vi "LinearQuadraticRegulator_Calculate.vi"(9 "X":T1, 11 "in LinearQuadraticRegulator":T2) -> (0 "Error":bool, 2 "U":T1, 3 "out LinearQuadraticRegulator":T2)   [LabVIEW 2019, in "Trajectory_Library.lvlib"]
doc: "Returns the next output of the controller.\n\nInputs:\n - LinearQuadraticRegulator -- controller data cluster \n - x -- The current state x.\n\nOutput:\n - outLinearQuadraticRegulator -- updated controller data cluster\n - U -- The next controller output.\n - error -- If TRUE, an error occured."
uses:
  Trajectory_Library.lvlib
  <vilib>/Analysis/NI_AALBase.lvlib
  <vilib>/Analysis/baseanly.llb/Real A x B.vi
  <vilib>/Analysis/Matrix/NI_Matrix.lvlib
  <vilib>/Analysis/Matrix/Numeric/Subtract/Subtract - RM,RM.vi
  <vilib>/Analysis/Matrix/Datatypes/RealMatrix.ctl
  TypeDef/LINEAR_QUADRATIC_REGULATOR.ctl
panel:
  # "Ref State <States,1>"
  # "Comp and capped \noutput <Inputs,1>"
  # "Controller gain\n<Inputs,States>"
  # "Ref State <States,1>"
  # "Comp and capped \noutput <Inputs,1>"
  # "Controller gain\n<Inputs,States>"
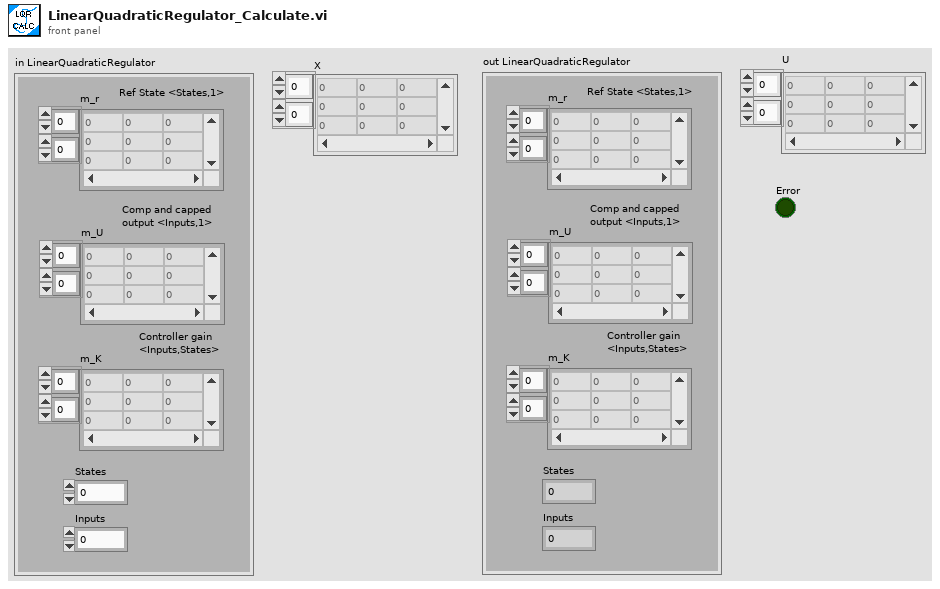
[diagram p1: front panel]
types:
  T1 = typedef "NI_Matrix.lvlib/RealMatrix.ctl" = dbl[][]
  T2 = typedef "Trajectory_Library.lvlib/LINEAR_QUADRATIC_REGULATOR.ctl" = cluster{"m_r":T1, "m_U":T1, "m_K":T1, "States":i32, "Inputs":i32}
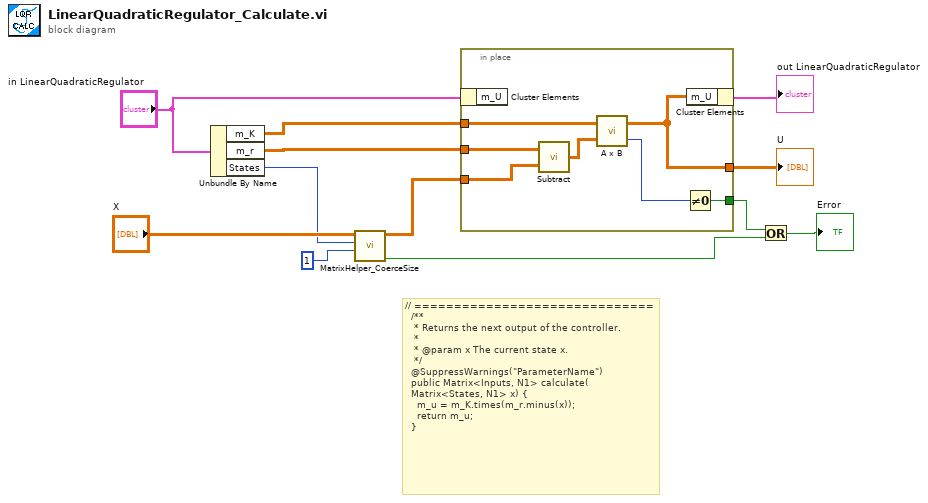
[diagram p0: block diagram]
diagram:
  # "// ==============================\n  /**\n   * Returns the next output of the controller.\n   *\n   * @param x The current state x.\n   */\n  @SuppressWarnings(\"ParameterName\")\n  public Matrix<Inputs, N1> calculate(\n\t\tMatrix<States, N1> x) {\n    m_u = m_K.times(m_r.minus(x));\n    return m_u;\n  }"
  n1 = Unbundle By Name("in LinearQuadraticRegulator") -> ("m_K"=w10:T1, "m_r"=w9:T1, "States"=w4:i32)
  n2 = call "MatrixHelper_CoerceSize.vi"("Columns"=1 ("y"), "Rows"=w4, "input matrix"="X") -> ("Coerced"=w1:bool, "output matrix"=w5:T1)  [unwired: 7 in]
  n3 = in-place {
    in-place-border: w10 -> [w19]
    in-place-border: w9 -> [w18]
    in-place-border: w5 -> [w17]
    in-place-border: [w15] -> w8
    in-place-border: [w13] -> w2
    n4 = in-place-cluster #1("in LinearQuadraticRegulator") -> ()  [unwired: 1 out]
    n5 = call-poly <vilib>:"Subtract.vi"("Real Matrix B"=w17, "Real Matrix A"=w18) -> ("A - B"=w16:T1)
    n6 = call-poly <vilib>:"A x B.vi"("B"=w16, "A"=w19) -> ("error"=w14:i32, "A x B"=w15:T1)
    n7 = Not Equal To 0?(x=w14) -> (x != 0?=w13:bool)
    n8 = in-place-cluster #1("m_U"=w15) -> (→"out LinearQuadraticRegulator":T2)
  }
  "U" <- w8
  n9 = Or(x=w2, y=w1) -> (x .or. y?=→"Error":bool)
